vi "FFT.vi"(8 "Error in":errorcluster, 9 "FFT size":i32=-1, 10 "Window":T1 items=["Rectangle", "Hanning", "Hamming", "Blackman-Harris", "Exact Blackman", "Blackman", "Flat Top", "4 Term B-Harris ", "7 Term B-Harris", "Low Sidelobe", "Blackman Nuttall", "Triangle", "Bartlett-Hanning", "Bohman", "Parzen", "Welch", "Kaiser", "Dolph-Chebyshev", "Gaussian"], 11 "Time Domain Signal":dbl[](array[numeric])) -> (0 "Error out":errorcluster, 3 "Frequency Domain Signal":dbl[](array[numeric]))   [LabVIEW 2021]
uses:
  <vilib>/Analysis/4window.llb/windowTd.ctl
  <vilib>/Analysis/0measdsp.llb/Scaled Time Domain Window (DBL).vi
  <vilib>/Analysis/NI_AALPro.lvlib
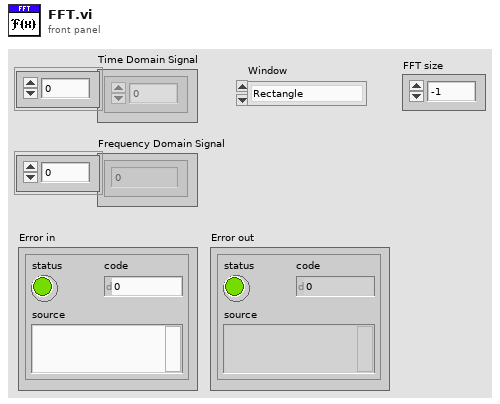
[diagram p1: front panel]
types:
  T1 = typedef "NI_AALPro.lvlib/windowTd.ctl" = u16
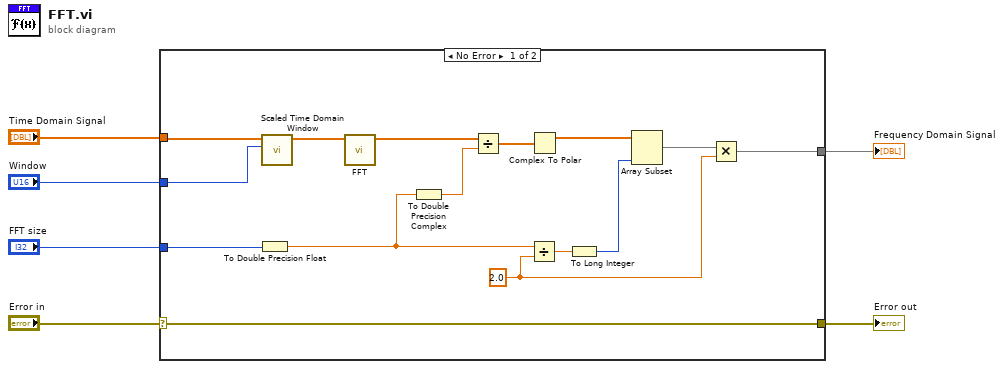
[diagram p0: block diagram]
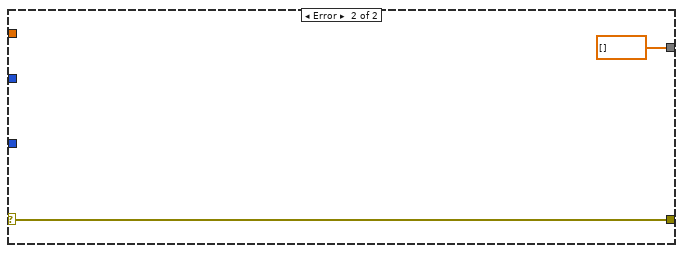
[diagram p2: hidden frame]
diagram:
  n1 = case shown="No Error" "Error in" {
    selector: "Error in" -> [w21 w23]
    tunnel: [w21 w23] -> w5
    tunnel: "Window" -> [w18 _]
    tunnel: "FFT size" -> [w14 _]
    tunnel: "Time Domain Signal" -> [w15 _]
    tunnel: [w9 dbl[] []] -> w1
    frame No Error {
      w8 = 2.0 ("y")
      n2 = To Double Precision Float(number=w14) -> (double precision float=w13:dbl)
      n3 = call-poly <vilib>:"Scaled Time Domain Window.vi"("window"=w18, "X"=w15) -> ("Windowed X"=w17:dbl[])  [unwired: 7 in, 2 out]
      n4 = call-poly <vilib>:"FFT.vi"("X"=w17) -> ("FFT {X}"=w7:cdb[])  [unwired: 9 in, 1 out]
      n5 = To Double Precision Complex(1:w13) -> (0:w12:cdb)
      n6 = Divide(x=w7, y=w12) -> (x/y=w19:cdb[])
      n7 = Divide(x=w13, y=w8) -> (x/y=w11:dbl)
      n8 = Complex To Polar(r * e^(i*theta)=w19) -> (r=w20:dbl[])  [unwired: 1 out]
      n9 = To Long Integer(number=w11) -> (32bit integer=w10:i32)
      n10 = Array Subset(array=w20, length=w10) -> (w16:dbl[])  [unwired: 1 in]
      n11 = Multiply(x=w16, y=w8) -> (x*y=w9:dbl[])
    }
    frame Error {
    }
  }
  "Error out" <- w5
  "Frequency Domain Signal" <- w1
